vi "Element Type.vi"(11 "NumericMatchBooleanIndicator in":refnum<class "NumericRangeBooleanIndicator.lvclass">) -> (2 "Element Type":string)   [LabVIEW 2020, in "VolatusGUIElements.lvlib" / "NumericRangeBooleanIndicator.lvclass"]
uses:
  NumericRangeBooleanIndicator.lvclass
  NumericRangeBooleanIndicator.lvclass/NumericRangeBooleanIndicator.ctl
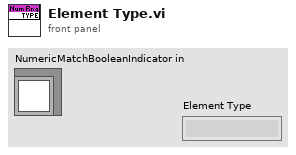
[diagram p1: front panel]
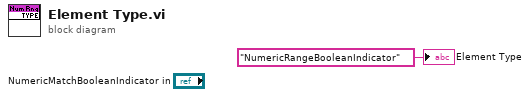
[diagram p0: block diagram]
diagram:
  "Element Type" <- "NumericRangeBooleanIndicator" ("Element Type")
